vi "servo.vi"(11 "Winkel soll":dbl) -> (3 "Winkel ist":dbl)   [LabVIEW 2019]
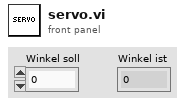
[diagram p1: front panel]
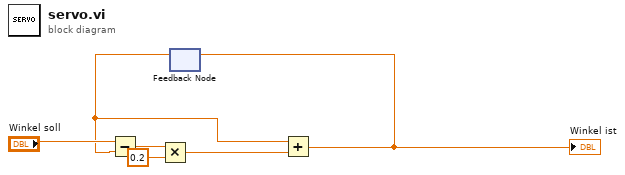
[diagram p0: block diagram]
diagram:
  n1 = feedback #1() -> (w1:dbl)  [unwired: 1 in]
  n2 = Subtract(x="Winkel soll", y=w1) -> (x-y=w4:dbl)
  n3 = Multiply(x=w4, y=0.2) -> (x*y=w2:dbl)
  n4 = Add(x=w1, y=w2) -> (x+y=w6:dbl)
  "Winkel ist" <- w6
  n5 = feedback-in #1(w6) -> ()
